vi "PPG_ABC.publish PGRunning.vi"(0 "i ref in":refnum<vi>, 2 "PPGRunning":T1, 3 "ms timeout (10000)":i32=10000, 5 "error in (no error)":errorcluster) -> (14 "i ref out":refnum<vi>, 17 "timed out":bool, 19 "error out":errorcluster)   [LabVIEW 2014, in "PPG_ABC.lvlib"]
doc: "Publishes the status of PPGRunning"
uses:
  PPG_ABC.lvlib
  PPG_ABC.PG_Running.ctl
  CSlibraries-extern/DimLVEvent/LVDimInterface/LVDimInterface.lvlib
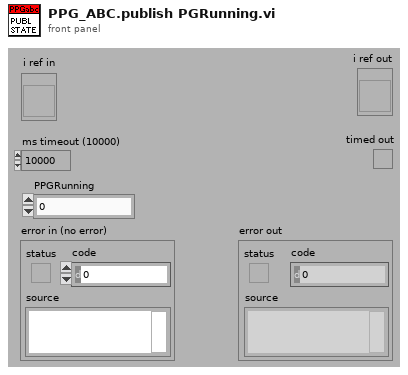
[diagram p1: front panel]
types:
  T1 = typedef "PPG_ABC.lvlib/PPG_ABC.PG_Running.ctl" = i32
  T2 = typedef "PPG_ABC.lvlib/PPG_ABC.i attribute.ctl" = cluster{"patternGroups":T3[], "defaultLetter":string, "defaultPatternGroup":i32, "PGRunning":T1, "PGRunningID":i32, "pgStarting":T4}
  T3 = typedef "PPG_ABC.lvlib/PPG_ABC.PG_dataType.ctl" = cluster{"PGDevice":string, "rawPatternData":cluster{"triggerCondition":i32, "timeTable":dbl[], "channelTable":string[]}[]}
  T4 = typedef "Semaphore RefNum" = refnum<k1>
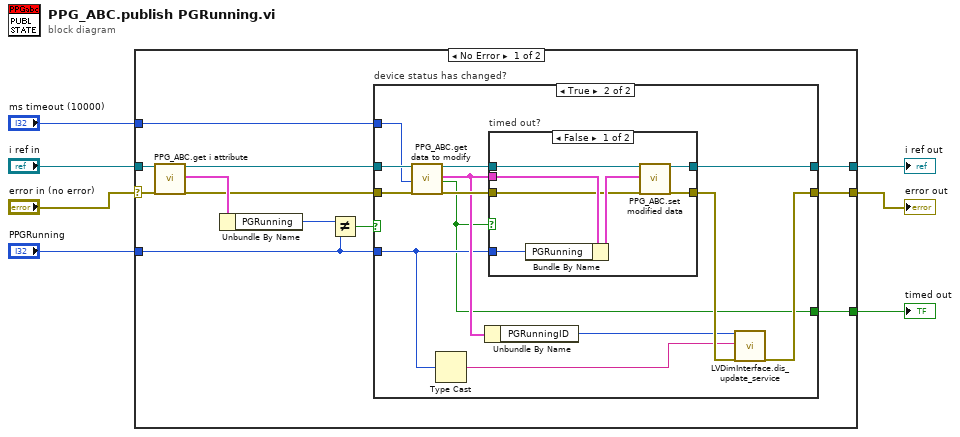
[diagram p0: block diagram]
diagram:
  n1 = case shown="No Error" "error in (no error)" {
    selector: "error in (no error)" -> [w11 w44]
    tunnel: "i ref in" -> [w12 w45]
    tunnel: [w14 w45] -> w5
    tunnel: [w13 w44] -> w4
    tunnel: "ms timeout (10000)" -> [w15 _]
    tunnel: "PPGRunning" -> [w9 _]
    tunnel: [w8 _] -> w1
    frame No Error {
      n2 = call "PPG_ABC.get i attribute.vi"("i ref in"=w12, "error in (no error)"=w11) -> ("i ref out"=w17:refnum<vi>, "i attribute"=w19:T2, "error out"=w16:errorcluster)  [unwired: 15 in]
      n3 = Unbundle By Name(w19) -> ("PGRunning"=w10:T1)
      n4 = Not Equal?(x=w10, y=w9) -> (x != y?=w18:bool)
      n5 = case "device status has changed?" shown="True" w18 {
        tunnel: w17 -> [w21 w34]
        tunnel: w16 -> [w20 w32]
        tunnel: w15 -> [_ w33]
        tunnel: [w21 w29] -> w14
        tunnel: [w20 w26] -> w13
        tunnel: w9 -> [_ w24]
        tunnel: [_ w22] -> w8
        frame False {
        }
        frame True {
          n6 = call "PPG_ABC.get data to modify.vi"("i ref in"=w34, "ms timeout (10000)"=w33, "error in (no error)"=w32) -> ("i ref out"=w31:refnum<vi>, "i attribute"=w28:T2, "timed out"=w22:bool, "error out"=w30:errorcluster)  [unwired: 13 in]
          n7 = Type Cast(x=w24) -> (*(type *) &x=w23:string)  [unwired: 1 in]
          n8 = Unbundle By Name(w28) -> ("PGRunningID"=w25:i32)
          n9 = case "timed out?" shown="False" w22 {
            tunnel: w31 -> [w36 w43]
            tunnel: w30 -> [w37 w42]
            tunnel: w28 -> [w39 _]
            tunnel: [w41 w43] -> w29
            tunnel: [w40 w42] -> w27
            tunnel: w24 -> [w35 _]
            frame False {
              n10 = Bundle By Name(cluster=w39, "PGRunning"=w35) -> (w38:T2)
              n11 = call "PPG_ABC.set modified data.vi"("i ref in"=w36, "i attribute"=w38, "error in (no error)"=w37) -> ("i ref out"=w41:refnum<vi>, "error out"=w40:errorcluster)  [unwired: 15 in]
            }
            frame True {
            }
          }
          n12 = call "LVDimInterface.dis_update_service.vi"("my_serviceID"=w25, "data"=w23, "error in (no error)"=w27) -> ("error out"=w26:errorcluster)  [unwired: 14 in, 2 out]
        }
      }
    }
    frame Error {
    }
  }
  "error out" <- w4
  "i ref out" <- w5
  "timed out" <- w1
